vi "Note Popup.vi"(9 "Main VI ref":refnum<vi>, 10 "SR Number":i32, 11 "File Loop Data":T1) -> ()   [LabVIEW 2018]
uses:
  Type Defs/File IO Loop Data.ctl
  Support/Message Queue/Message Cluster.ctl
  <vilib>/Utility/miscctls.llb/LVSelectionTypeDef.ctl
  Support/Message Queue/Enqueue Message (Single).vi
  Support/Message Queue/Message Queue.lvlib
panel:
  in  "Cancel Button":bool
  in  "Save Button":bool
  in  "Notes":string
  in  "Error In":errorcluster
  out "Help Text":string
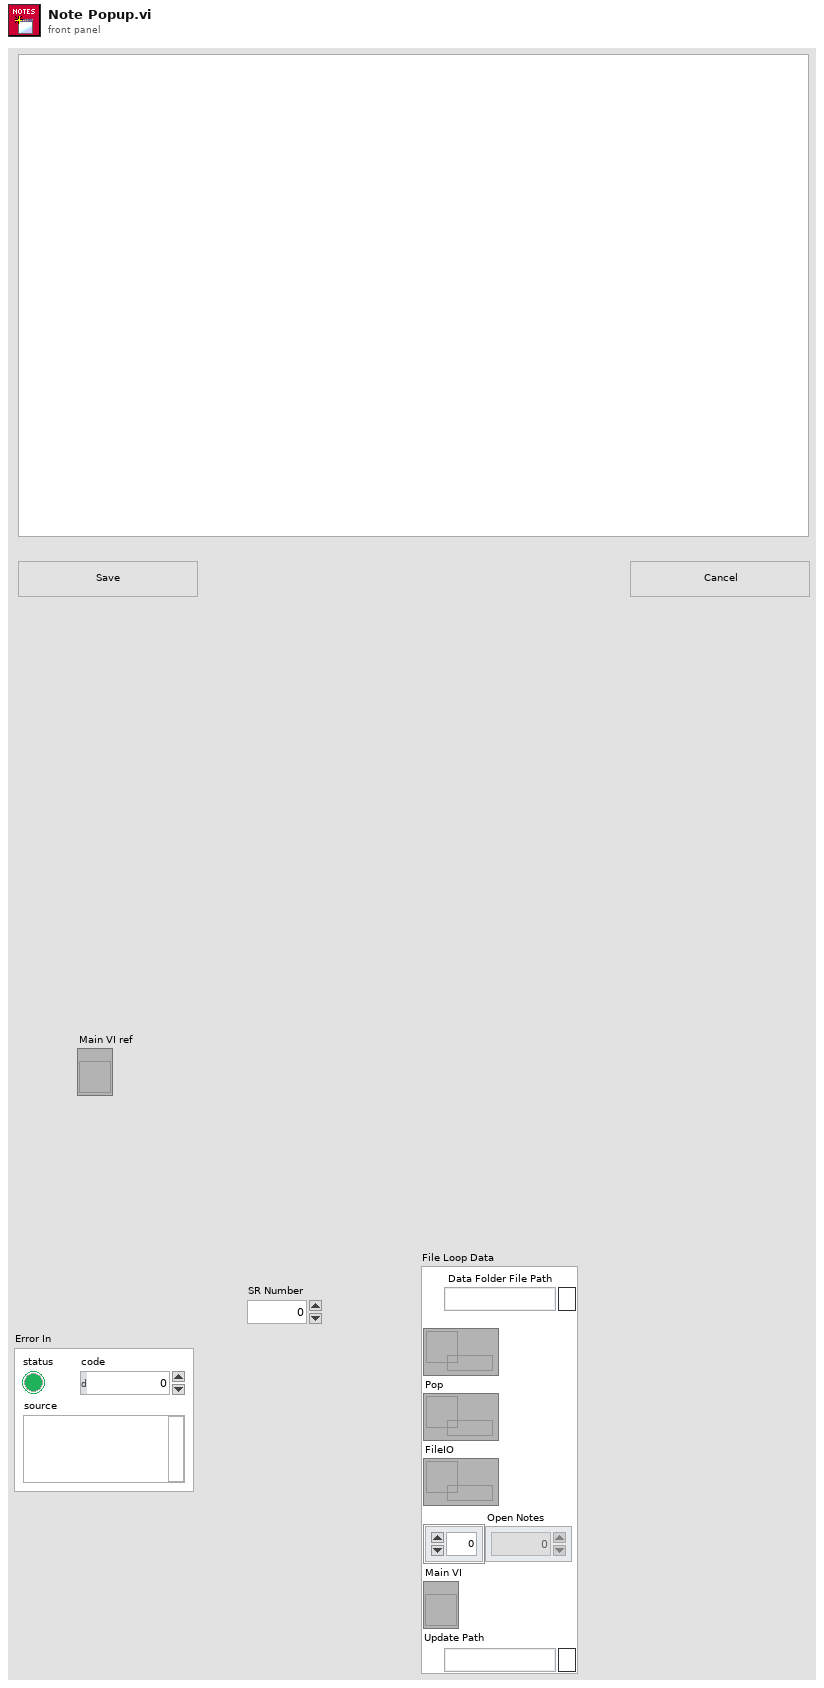
[diagram p1: front panel]
types:
  T1 = typedef "File IO Loop Data.ctl" = cluster{"Data Folder File Path":path, "UI":refnum<queue>, "Pop":refnum<queue>, "FileIO":refnum<queue>, "Open Notes":i32[], "Main VI":refnum<vi>, "Update Path":path}
  T2 = typedef "LVSelectionTypeDef.ctl" = cluster{"Selection Start":u32, "Selection End":u32}
  T3 = enum16{"Left Button", "Center Button", "Right Button", "Window Close"}
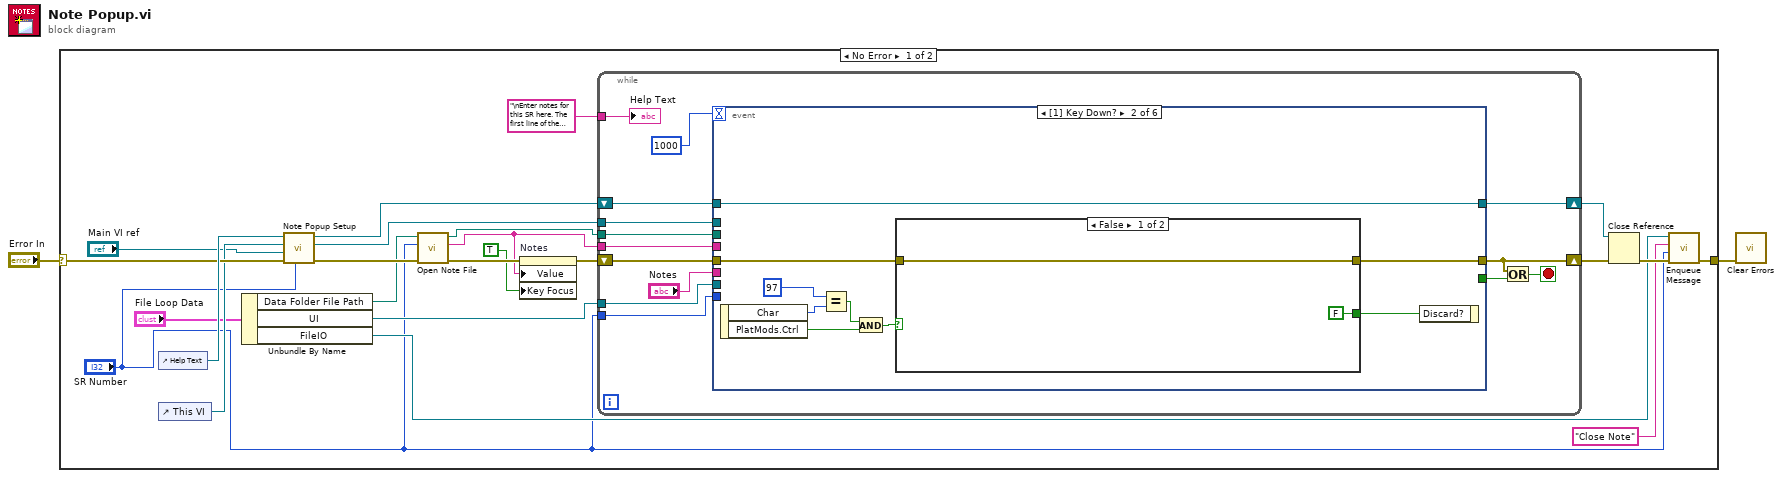
[diagram p0: block diagram]
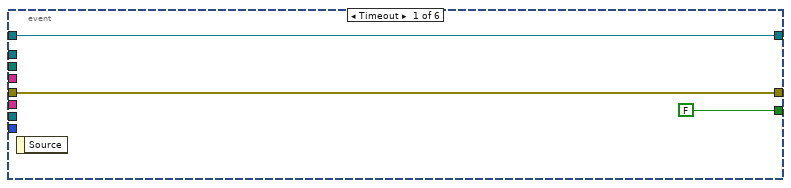
[diagram p2: hidden frame]
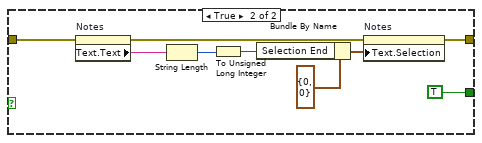
[diagram p3: hidden frame]
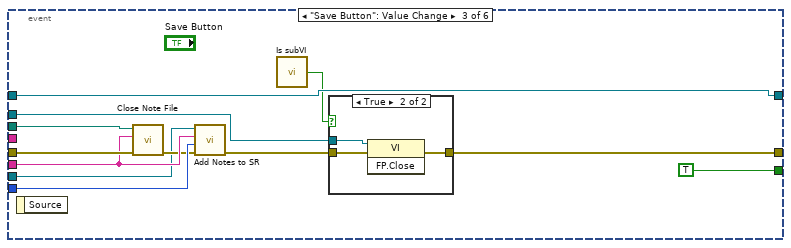
[diagram p4: hidden frame]
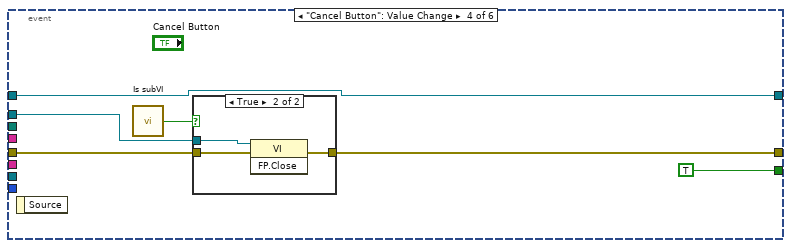
[diagram p6: hidden frame]
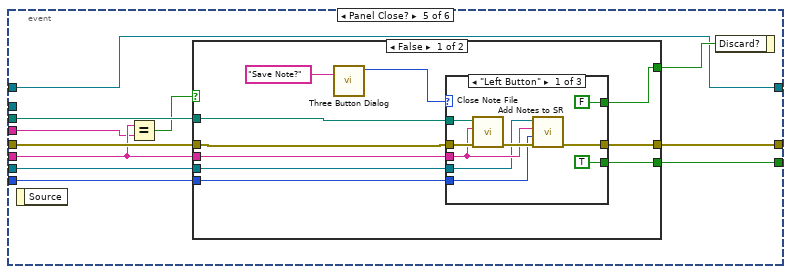
[diagram p8: hidden frame]
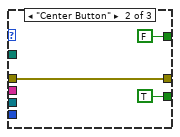
[diagram p9: hidden frame]
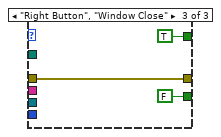
[diagram p10: hidden frame]
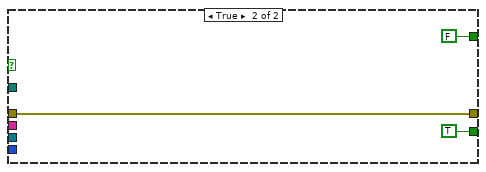
[diagram p11: hidden frame]
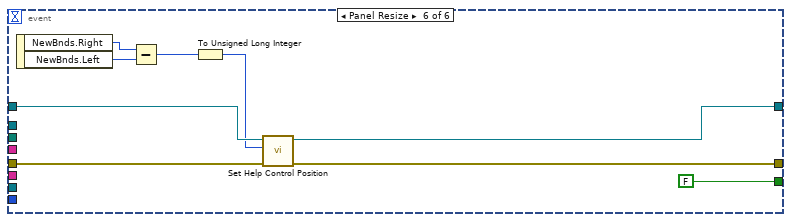
[diagram p12: hidden frame]
diagram:
  n1 = case shown="No Error" "Error In" {
    selector: "Error In" -> [w18 w137]
    tunnel: [w11 w137] -> w1
    frame No Error {
      n2 = control-ref of="Help Text"() -> (w21:refnum<vi>)
      n3 = control-ref of="This VI"() -> (w10:refnum<vi>)
      n4 = Unbundle By Name("File Loop Data") -> ("Data Folder File Path"=w7:path, "UI"=w14:refnum<queue>, "FileIO"=w12:refnum<queue>)
      n5 = call "Note Popup Setup.vi"("SR Number"="SR Number", "error in"=w18, "Main VI ref in"="Main VI ref", "This VI in"=w10, "string ref in"=w21) -> ("error out"=w19:errorcluster, "This VI out"=w15:refnum<vi>, "string ref out"=w20:refnum<vi>)  [unwired: 3 in, 1 out]
      n6 = call "Open Note File.vi"("Error In"=w19, "SR Number"="SR Number", "Folder path"=w7) -> ("Error Out"=w24:errorcluster, "Notes"=w3:string, "file path"=w25:path)  [unwired: 6 in]
      n7 = property on="Notes" class="Str"(error in=w24, "Value"=w3, "Key Focus"=TRUE) -> (error out=w23:errorcluster)  [unwired: 1 in, 1 out]
      n8 = while {
        tunnel: w25 -> [w36]
        shift-right: [w33] -> w16
        shift-left: w23 -> [w38]
        tunnel: "\nEnter notes for this SR here. The first line of the entered text will be displayed on the front panel." ("Help Text") -> [w32]
        shift-right: [w30] -> w17
        shift-left: w20 -> [w31]
        tunnel: "SR Number" -> [w29]
        tunnel: w15 -> [w28]
        tunnel: w14 -> [w27]
        tunnel: w3 -> [w26]
        stop <- w35 stop-if-true
        n9 = event shown="[1] Key Down?" {
          selector: _ -> [_ _ _ _ _ _]
          dyn-events: _ -> [_ _ _ _ _ _]
          timeout: 1000 -> [_ _ _ _ _ _]
          tunnel: [FALSE _ TRUE TRUE w99 FALSE] -> w34
          tunnel: w38 -> [w41 w46 w73 w82 w98 w133]
          tunnel: [w41 w45 w65 w81 w97 w132] -> w33
          tunnel: "Notes" -> [_ _ w70 _ w91 _]
          tunnel: w36 -> [_ _ w72 _ w96 _]
          tunnel: w31 -> [w40 w51 w71 w83 w92 w130]
          tunnel: [w40 w51 w71 w83 w92 w131] -> w30
          tunnel: w29 -> [_ _ w69 _ w95 _]
          tunnel: w28 -> [_ _ w67 w80 _ _]
          tunnel: w27 -> [_ _ w63 _ w93 _]
          tunnel: w26 -> [_ _ _ _ w90 _]
          event Timeout {
            n10 = event-data() -> ()  [unwired: 1 in, 1 out]
          }
          event Key Down? {
            n11 = event-data() -> ("Char"=w50:i16, "PlatMods.Ctrl"=w47:bool)  [unwired: 1 in]
            n12 = Equal?(x=i16 97, y=w50) -> (x = y?=w48:bool)
            n13 = And(x=w48, y=w47) -> (x .and. y?=w44:bool)
            n14 = case shown="False" w44 {
              tunnel: w46 -> [w53 w60]
              tunnel: [w53 w62] -> w45
              tunnel: [FALSE ("Discard?") TRUE ("Discard?")] -> w43
              frame False {
              }
              frame True {
                n15 = property on="Notes" class="Str"(error in=w60) -> (error out=w58:errorcluster, "Text.Text"=w55:string)  [unwired: 1 in, 1 out]
                n16 = String Length(string=w55) -> (length=w57:i32)
                n17 = To Unsigned Long Integer(number=w57) -> (unsigned 32bit integer=w56:u32)
                n18 = Bundle By Name(cluster=T2 {"Selection Start"=0, "Selection End"=0} ("Text.Selection"), "Selection End"=w56) -> (w59:T2)
                n19 = property on="Notes" class="Str"(error in=w58, "Text.Selection"=w59) -> (error out=w62:errorcluster)  [unwired: 1 in, 1 out]
              }
            }
            n20 = event-data("Discard?"=w43) -> ()  [unwired: 1 in, 1 out]
          }
          event "Save Button": Value Change {
            n21 = event-data() -> ()  [unwired: 1 in, 1 out]
            n22 = call "Close Note File.vi"("Error In"=w73, "Notes"=w70, "file path"=w72) -> ("Error Out"=w68:errorcluster)  [unwired: 8 in]
            n23 = call "Add Notes to SR.vi"("Error In"=w68, "SR Number"=w69, "Note to Add"=w70, "UI"=w63) -> ("Error Out"=w66:errorcluster)  [unwired: 7 in]
            n24 = call "Is subVI.vi"() -> ("Is subVI?"=w64:bool)  [unwired: 1 in]
            n25 = case shown="True" w64 {
              tunnel: w67 -> [_ w78]
              tunnel: w66 -> [w75 w77]
              tunnel: [w75 w76] -> w65
              frame False {
              }
              frame True {
                n26 = invoke class="VI" method="FP.Close"(reference=w78, error in=w77) -> (error out=w76:errorcluster)  [unwired: 1 in, 2 out]
              }
            }
          }
          event "Cancel Button": Value Change {
            n27 = event-data() -> ()  [unwired: 1 in, 1 out]
            n28 = call "Is subVI.vi"() -> ("Is subVI?"=w79:bool)  [unwired: 1 in]
            n29 = case shown="True" w79 {
              tunnel: w82 -> [w85 w88]
              tunnel: [w85 w87] -> w81
              tunnel: w80 -> [_ w86]
              frame False {
              }
              frame True {
                n30 = invoke class="VI" method="FP.Close"(reference=w86, error in=w88) -> (error out=w87:errorcluster)  [unwired: 1 in, 2 out]
              }
            }
          }
          event Panel Close? {
            n31 = event-data() -> ()  [unwired: 1 in, 1 out]
            n32 = Equal?(x=w91, y=w90) -> (x = y?=w89:bool)
            n33 = case shown="False" w89 {
              tunnel: [w108 TRUE] -> w99
              tunnel: w98 -> [w107 w126]
              tunnel: [w106 w126] -> w97
              tunnel: w91 -> [w105 _]
              tunnel: w96 -> [w103 _]
              tunnel: w95 -> [w100 _]
              tunnel: [w102 FALSE ("Discard?")] -> w94
              tunnel: w93 -> [w101 _]
              frame False {
                n34 = call <vilib>:"Three Button Dialog.vi"("message"="Save Note?") -> ("Which Button?"=w104:T3)  [unwired: 10 in]
                n35 = case shown="\"Left Button\"" w104 {
                  tunnel: [FALSE ("Discard?") FALSE ("Discard?") TRUE ("Discard?")] -> w102
                  tunnel: [TRUE TRUE FALSE] -> w108
                  tunnel: w107 -> [w116 w119 w122]
                  tunnel: [w114 w119 w122] -> w106
                  tunnel: w105 -> [w111 _ _]
                  tunnel: w103 -> [w115 _ _]
                  tunnel: w100 -> [w112 _ _]
                  tunnel: w101 -> [w110 _ _]
                  frame "Left Button" {
                    n36 = call "Close Note File.vi"("Error In"=w116, "Notes"=w111, "file path"=w115) -> ("Error Out"=w113:errorcluster)  [unwired: 8 in]
                    n37 = call "Add Notes to SR.vi"("Error In"=w113, "SR Number"=w112, "Note to Add"=w111, "UI"=w110) -> ("Error Out"=w114:errorcluster)  [unwired: 7 in]
                  }
                  frame "Center Button" {
                  }
                  frame "Right Button", "Window Close" {
                  }
                }
              }
              frame True {
              }
            }
            n38 = event-data("Discard?"=w94) -> ()  [unwired: 1 in, 1 out]
          }
          event Panel Resize {
            n39 = event-data() -> ("NewBnds.Right"=w135:i16, "NewBnds.Left"=w134:i16)  [unwired: 1 in]
            n40 = Subtract(x=w135, y=w134) -> (x-y=w129:i16)
            n41 = To Unsigned Long Integer(number=w129) -> (unsigned 32bit integer=w128:u32)
            n42 = call "Set Help Control Position.vi"("error in (no error)"=w133, "Width"=w128, "String in"=w130) -> ("error out"=w132:errorcluster, "String out"=w131:refnum<vi>)  [unwired: 7 in]
          }
        }
        n43 = Or(x=w33, y=w34) -> (x .or. y?=w35:bool)
        "Help Text" <- w32
      }
      n44 = Close Reference(reference=w17, error in (no error)=w16) -> (error out=w13:errorcluster)
      n45 = call-poly "Enqueue Message.vi"("error in (no error)"=w13, "Message Data"="SR Number", "Message"="Close Note", "Message Queue"=w12) -> ("error out"=w11:errorcluster)  [unwired: 6 in, 1 out]
    }
    frame Error {
    }
  }
  n46 = call <vilib>:"Clear Errors.vi"("error in (no error)"=w1) -> ()  [unwired: 5 in, 2 out]
